vi "Wiimote Open.vi"(8 "error in":errorcluster, 11 "index":i32) -> (0 "error out":errorcluster, 3 "hWiimoteHandle":u32 format="%08x")   [LabVIEW 2012, in "Wiimote.lvlib"]
uses:
  Wiimote.lvlib
  wiimote.dll
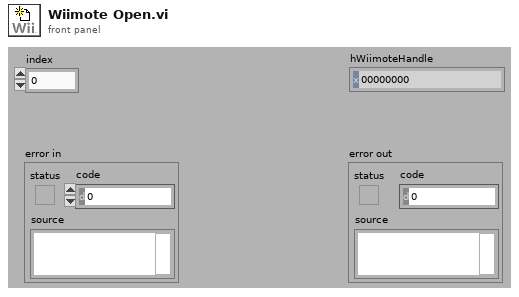
[diagram p1: front panel]
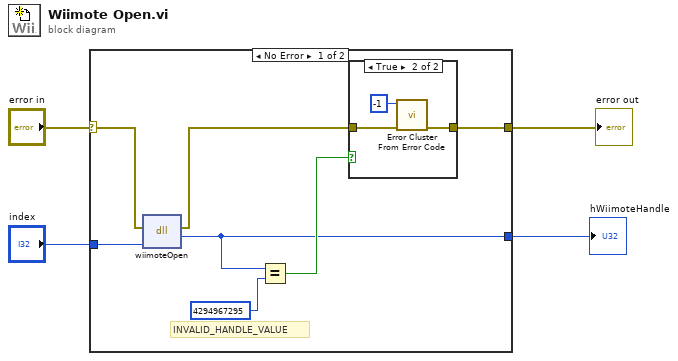
[diagram p0: block diagram]
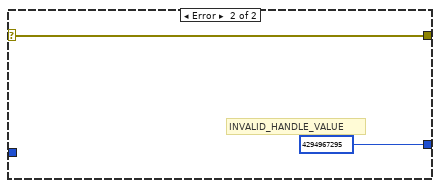
[diagram p3: hidden frame]
diagram:
  n1 = case shown="No Error" "error in" {
    selector: "error in" -> [w7 w17]
    tunnel: [w11 w17] -> w3
    tunnel: [w5 u32 4294967295 ("hWiimoteHandle")] -> w2
    tunnel: "index" -> [w6 _]
    frame No Error {
      # "INVALID_HANDLE_VALUE"
      n2 = dll-call lib="C:/Users/whitemrj/Documents/GitHub/IGVC-2013/Code/Project 1.0/Remotes/Wiimote/Wiimote/wiimote.dll" fn="wiimoteOpen"(error in=w7, "index"=w6) -> (error out=w8:errorcluster, "return type"=w5:u32)  [unwired: 3 in, 1 out]
      n3 = Equal?(x=w5, y=u32 4294967295 ("hWiimoteHandle")) -> (x = y?=w9:bool)
      n4 = case shown="True" w9 {
        tunnel: [w12 w15] -> w11
        tunnel: w8 -> [w12 w13]
        frame False {
        }
        frame True {
          n5 = call <vilib>:"Error Cluster From Error Code.vi"("error in (no error)"=w13, "error code (0)"=-1) -> ("error out"=w15:errorcluster)  [unwired: 7 in]
        }
      }
    }
    frame Error {
      # "INVALID_HANDLE_VALUE"
    }
  }
  "error out" <- w3
  "hWiimoteHandle" <- w2
